vi "SUB_SoundCard_DTMF_Decoder.vi"() -> ()   [LabVIEW 2011]
doc: "This example shows how to construct a simple Spectrum Analyzer example using the EASY I/O Sound VIs and the MEASUREMENT VIs. This example acquires a waveform, windows it, computes the autopower spectrum and the power and frequency of the peak frequency component. The power spectrum is graphed in the desired units."
uses:
  <vilib>/sound/lvsound.llb/Sound Format.ctl
  <vilib>/Analysis/NI_AALPro.lvlib
panel:
  in  "stop":bool
  in  "clear":bool
  out "Detected Numbers":string
  out "high tone":dbl
  out "low tone":dbl
  out "error in (no error)":errorcluster
  # "82102 DTMF Decoder 代刚"
  # "Detected Tones"
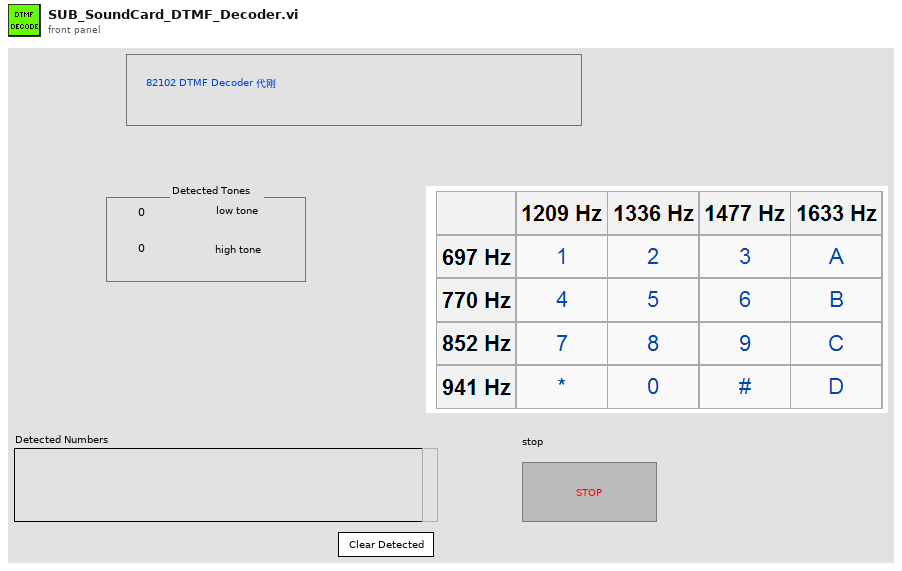
[diagram p1: front panel]
types:
  T1 = typedef "Sound Format.ctl" = cluster{"sound quality":enum16{"mono", "stereo"}, "rate":enum16{"11025", "22050", "44100", "8000"}, "bits per sample":enum16{"8 bit", "16 bit"}}
  T2 = enum32{"Lowpass", "Highpass", "Bandpass", "Bandstop"}
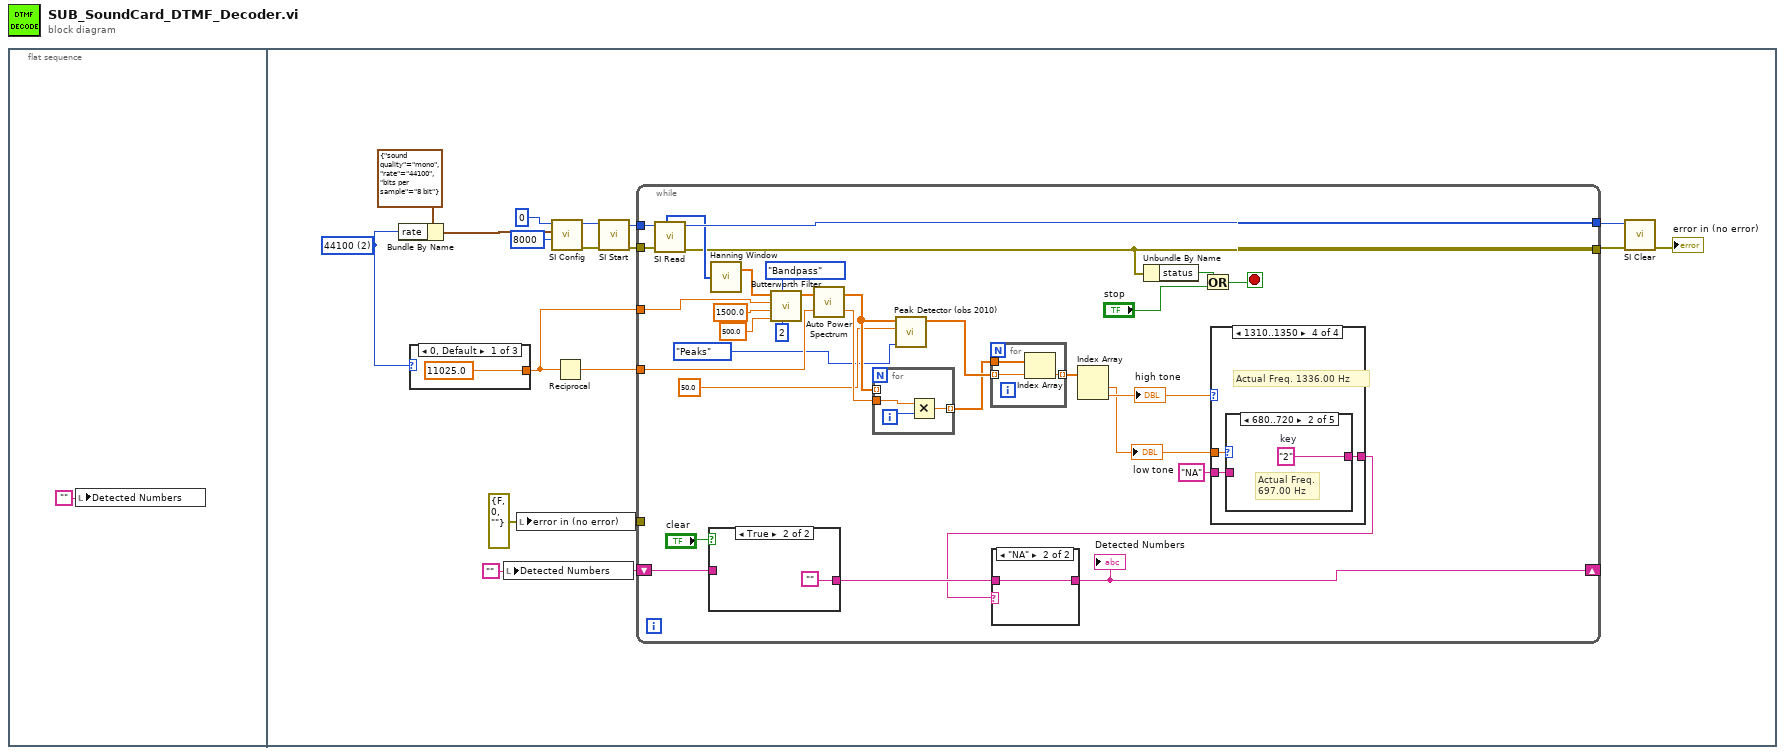
[diagram p0: block diagram]
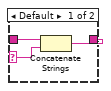
[diagram p3: hidden frame]
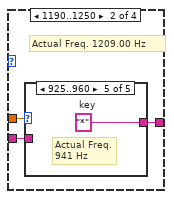
[diagram p5: hidden frame]
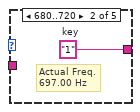
[diagram p7: hidden frame]
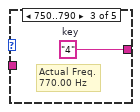
[diagram p8: hidden frame]
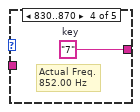
[diagram p9: hidden frame]
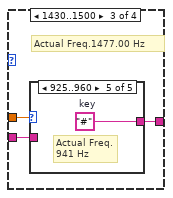
[diagram p10: hidden frame]
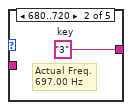
[diagram p12: hidden frame]
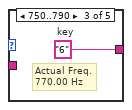
[diagram p13: hidden frame]
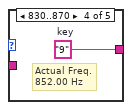
[diagram p14: hidden frame]
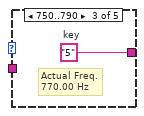
[diagram p16: hidden frame]
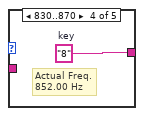
[diagram p17: hidden frame]
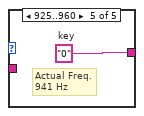
[diagram p18: hidden frame]
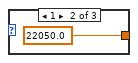
[diagram p19: hidden frame]
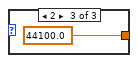
[diagram p20: hidden frame]
diagram:
  n1 = flat-sequence {
    frame #0 {
      n2 = local write "Detected Numbers"("") -> ()
    }
    frame #1 {
      w17 = u16 2 items=["11025", "22050", "44100"] ("Sample Rate")
      w4 = errorcluster {"status"=FALSE, "code"=0, "source"=""} ("error in (no error)")
      w6 = ""
      n3 = Bundle By Name(cluster=T1 {"sound quality"=enum."mono", "rate"=enum."44100", "bits per sample"=enum."8 bit"} ("sound format"), "rate"=w17) -> (w13:T1)
      n4 = case shown="0, Default" w17 {
        tunnel: [11025.0 22050.0 44100.0] -> w14
        frame 0, Default {
        }
        frame 1 {
        }
        frame 2 {
        }
      }
      n5 = local write "Detected Numbers"(w6) -> ()
      n6 = local write "error in (no error)"(w4) -> ()
      n7 = call <vilib>:"SI Config.vi"("buffer size (8192 in bytes)"=u32 8000, "sound format"=w13, "device (0)"=u32 0) -> ("error out"=w11:errorcluster, "task ID out"=w12:u32)  [unwired: 7 in]
      n8 = Reciprocal(x=w14) -> (1/x=w15:dbl)
      n9 = call <vilib>:"SI Start.vi"("error in (no error)"=w11, "task ID in"=w12) -> ("error out"=w9:errorcluster, "task ID out"=w10:u32)  [unwired: 8 in]
      n10 = while {
        tunnel: w15 -> [w48]
        tunnel: w14 -> [w35]
        tunnel: w10 -> [w44]
        tunnel: w9 -> [w43]
        tunnel: [w24] -> w8
        tunnel: [w42] -> w7
        shift-right: [w28] -> _
        shift-left: w6 -> [w25]
        tunnel: w4 -> [_]
        stop <- w22 stop-if-true
        n11 = call <vilib>:"SI Read.vi"("error in (no error)"=w43, "task ID in"=w44) -> ("error out"=w24:errorcluster, "task ID out"=w42:u32, "mono 8-bit"=w34:u8[])  [unwired: 4 in, 3 out]
        n12 = case shown="True" "clear" {
          tunnel: [w49 ""] -> w26
          tunnel: w25 -> [w49 _]
          frame False {
          }
          frame True {
          }
        }
        n13 = call "Hanning Window.vi"("X"=w34) -> ("Hanning {X}"=w36:dbl[])  [unwired: 1 out]
        n14 = call "Butterworth Filter.vi"("order"=2, "filter type"=T2."Bandpass", "low cutoff freq: fl"=500.0, "high cutoff freq: fh"=1500.0, "sampling freq: fs"=w35, "X"=w36) -> ("Filtered X"=w45:dbl[])  [unwired: 2 in, 1 out]
        n15 = call "Auto Power Spectrum.vi"("dt"=w48, "Signal (V)"=w45) -> ("df"=w30:dbl, "Power Spectrum (V^2 rms)"=w29:dbl[])
        n16 = for {
          tunnel: w30 -> [w81]
          tunnel: [w80] -> w40 mode=indexing
          tunnel: w29 -> [_] mode=indexing
          i -> [w82]
          n17 = Multiply(x=w81, y=w82) -> (x*y=w80:dbl)
        }
        n18 = call <vilib>:"Peak Detector (obs 2010).vi"("peaks/valleys"=enum32{"Peaks", "Valleys"}."Peaks", "threshold"=50.0, "X"=w29) -> ("Locations"=w41:dbl[])  [unwired: 4 in, 4 out]
        n19 = for {
          tunnel: w41 -> [w84] mode=indexing
          tunnel: w40 -> [w85]
          tunnel: [w83] -> w39 mode=indexing
          n20 = Index Array(array=w85, index=w84) -> (element=w83:dbl)
        }
        n21 = Index Array(array=w39) -> (element #1=w32:dbl, element #2=w33:dbl)  [unwired: 2 in]
        "low tone" <- w32
        "high tone" <- w33
        n22 = Unbundle By Name(w24) -> ("status"=w23:bool)
        n23 = Or(x=w23, y="stop") -> (x .or. y?=w22:bool)
        n24 = case shown="1310..1350" w33 {
          tunnel: w32 -> [_ w58 w66 w74]
          tunnel: [w55 w57 w65 w73] -> w21
          tunnel: "NA" ("Button") -> [w55 w56 w64 w72]
          frame Default {
          }
          frame 1190..1250 {
            # "Actual Freq. 1209.00 Hz"
            n25 = case shown="925..960" w58 {
              tunnel: [w59 w60 w61 w62 w63] -> w57
              tunnel: w56 -> [w59 _ _ _ _]
              frame Default {
              }
              frame 680..720 {
                w60 = "1"  # key
                # "Actual Freq. 697.00 Hz"
              }
              frame 750..790 {
                w61 = "4"  # key
                # "Actual Freq. 770.00 Hz"
              }
              frame 830..870 {
                w62 = "7"  # key
                # "Actual Freq. 852.00 Hz"
              }
              frame 925..960 {
                w63 = "*"  # key
                # "Actual Freq. 941 Hz"
              }
            }
          }
          frame 1430..1500 {
            # "Actual Freq.1477.00 Hz"
            n26 = case shown="925..960" w66 {
              tunnel: [w67 w68 w69 w70 w71] -> w65
              tunnel: w64 -> [w67 _ _ _ _]
              frame Default {
              }
              frame 680..720 {
                w68 = "3"  # key
                # "Actual Freq. 697.00 Hz"
              }
              frame 750..790 {
                w69 = "6"  # key
                # "Actual Freq. 770.00 Hz"
              }
              frame 830..870 {
                w70 = "9"  # key
                # "Actual Freq. 852.00 Hz"
              }
              frame 925..960 {
                w71 = "#"  # key
                # "Actual Freq. 941 Hz"
              }
            }
          }
          frame 1310..1350 {
            # "Actual Freq. 1336.00 Hz"
            n27 = case shown="680..720" w74 {
              tunnel: [w75 w76 w77 w78 w79] -> w73
              tunnel: w72 -> [w75 _ _ _ _]
              frame Default {
              }
              frame 680..720 {
                w76 = "2"  # key
                # "Actual Freq. 697.00 Hz"
              }
              frame 750..790 {
                w77 = "5"  # key
                # "Actual Freq. 770.00 Hz"
              }
              frame 830..870 {
                w78 = "8"  # key
                # "Actual Freq. 852.00 Hz"
              }
              frame 925..960 {
                w79 = "0"  # key
                # "Actual Freq. 941 Hz"
              }
            }
          }
        }
        n28 = case shown="\"NA\"" w21 {
          selector: w21 -> [w51 _]
          tunnel: w26 -> [w53 w54]
          tunnel: [w52 w54] -> w28
          frame Default {
            n29 = Concatenate Strings(w53, w51) -> (w52:string)
          }
          frame "NA" {
          }
        }
        "Detected Numbers" <- w28
      }
      n30 = call <vilib>:"SI Clear.vi"("error in (no error)"=w8, "task ID in"=w7) -> ("error out"=→"error in (no error)":errorcluster)  [unwired: 9 in]
    }
  }
